vi "Calculate Padding Buffer Size.vi"(10 "LP  F":dbl=0.001 format="%#_6p", 11 "Array size":i32) -> (1 "Last element":i32, 2 "First element":i32, 3 "Buffer size":i32)   [LabVIEW 2019]
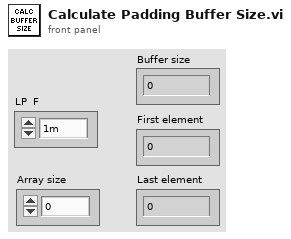
[diagram p1: front panel]
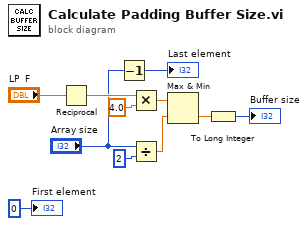
[diagram p0: block diagram]
diagram:
  n1 = Reciprocal(x="LP  F") -> (1/x=w9:dbl)
  n2 = Decrement(x="Array size") -> (x-1=→"Last element":i32)
  n3 = Multiply(x=w9, y=4.0) -> (x*y=w10:dbl)
  n4 = Divide(x="Array size", y=2) -> (x/y=w2:dbl)
  n5 = Max & Min(x=w10, y=w2) -> (min(x,y)=w7:dbl)  [unwired: 1 out]
  n6 = To Long Integer(number=w7) -> (32bit integer=→"Buffer size":i32)
  "First element" <- 0 ("First element")
